vi "Simulate Front Panel Key Press.vi"(8 "error in (no error)":errorcluster, 10 "Front Panel Key (Down Cursor)":T1, 11 "VISA resource name":refnum<visa-resource-name>) -> (0 "error out":errorcluster, 3 "VISA resource name out":refnum<visa-resource-name>)   [LabVIEW 2013, in "SRS SR400.lvlib"]
doc: "<B>CK j</B>\n\nThe CK command simulates pressing a front panel key. j is a required parameter from 0 to 13. The CK command may be sent at any time and is not restricted by the remote/local state of the front panel.\n\n<B>j</B> <B>key</B>\n0 DOWN CURSOR\n1 RIGHT CURSOR\n2 LEVEL\n3 SETUP\n4 COM\n5 STOP\n6 LOCAL\n7 RESET\n8 LEFT CURSOR\n9 UP CURSOR\n10 MODE\n11 AGATE\n12 BGATE\n13 START"
uses:
  <instrlib>/SRS SR400/SRS SR400.lvlib
  <instrlib>/SRS SR400/Public/Typedefs/Front Panel Key.ctl
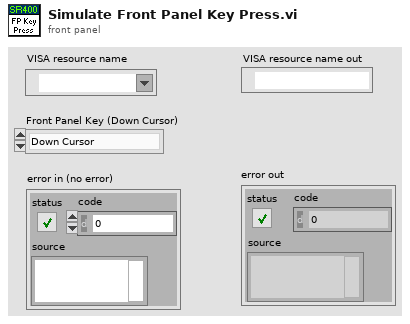
[diagram p1: front panel]
types:
  T1 = typedef "SRS SR400.lvlib/Front Panel Key.ctl" = enum16{"Down Cursor", "Right Cursor", "Level", "Setup", "Com", "Stop", "Local", "Reset", "Left Cursor", "Up Cursor", "Mode", "A Gate", "B Gate", "Start"}
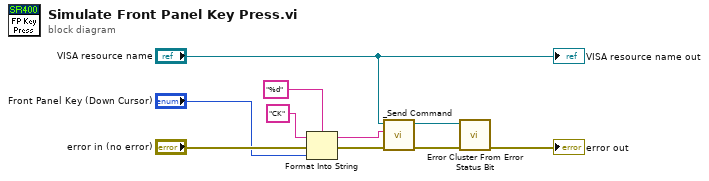
[diagram p0: block diagram]
diagram:
  n1 = Format Into String(format string="%d", initial string="CK" ("command"), error in="error in (no error)", "Front Panel Key (Down Cursor)") -> (resulting string=w7:string, error out=w6:errorcluster)
  n2 = call <instrlib>:"_Send Command.vi"("error in (no error)"=w6, "Command"=w7, "VISA resource name"="VISA resource name") -> ("error out"=w2:errorcluster, "VISA resource name out"=w3:refnum<visa-resource-name>)  [unwired: 1 in, 6 out]
  n3 = call <instrlib>:"Error Cluster From Error Status Bit.vi"("error in (no error)"=w2, "VISA resource name"=w3) -> ("error out"=→"error out":errorcluster)  [unwired: 8 in, 1 out]
  "VISA resource name out" <- "VISA resource name"
